vi "Plugin - Mid Measurement.vi"(11 "Message Queues in":T1) -> ()   [LabVIEW 2019]
uses:
  support/Copy of Message Queue/All Message Queues.ctl
  support/Copy of Message Queue/Message Cluster.ctl
  Analysis/Global Tube Measurement.vi
  support/Message Queue/Message Queue.lvlib
  support/Copy of Message Queue/Copy of Message Queue.lvlib
panel:
  in  "Mid Measurement(m)":dbl format="%.4g"
  in  "error in":errorcluster
  out "error out":errorcluster
  in  "Next":bool
  in  "Exit":bool
  # "Enter Mid Measurement"
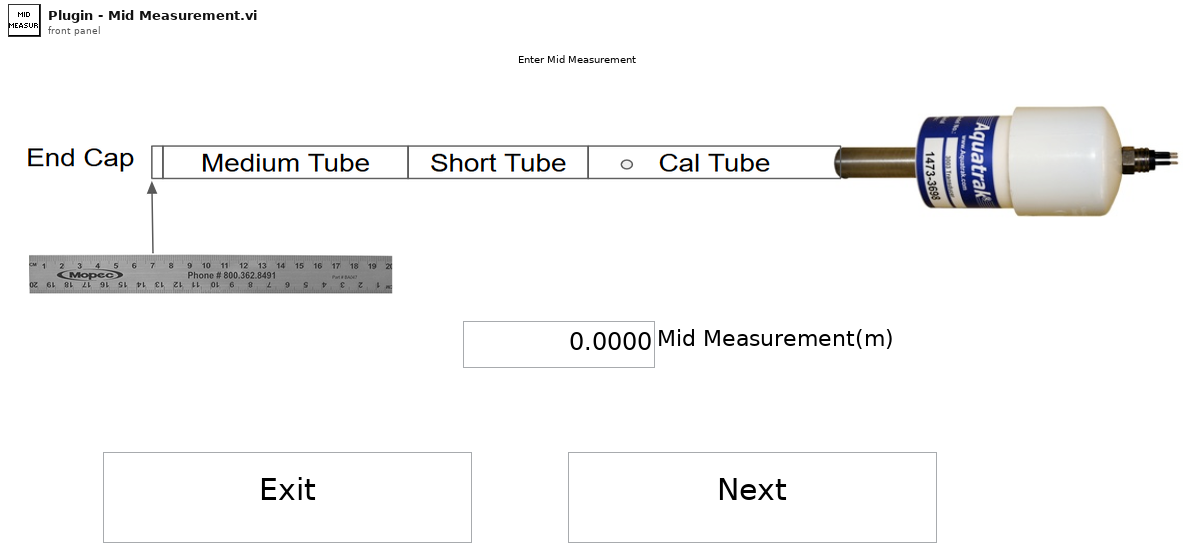
[diagram p1: front panel]
types:
  T1 = typedef "Copy of Message Queue.lvlib/All Message Queues.ctl" = cluster{"UI":refnum<queue>, "Acquisition":refnum<queue>, "Logging":refnum<queue>, "Analyze":refnum<queue>}
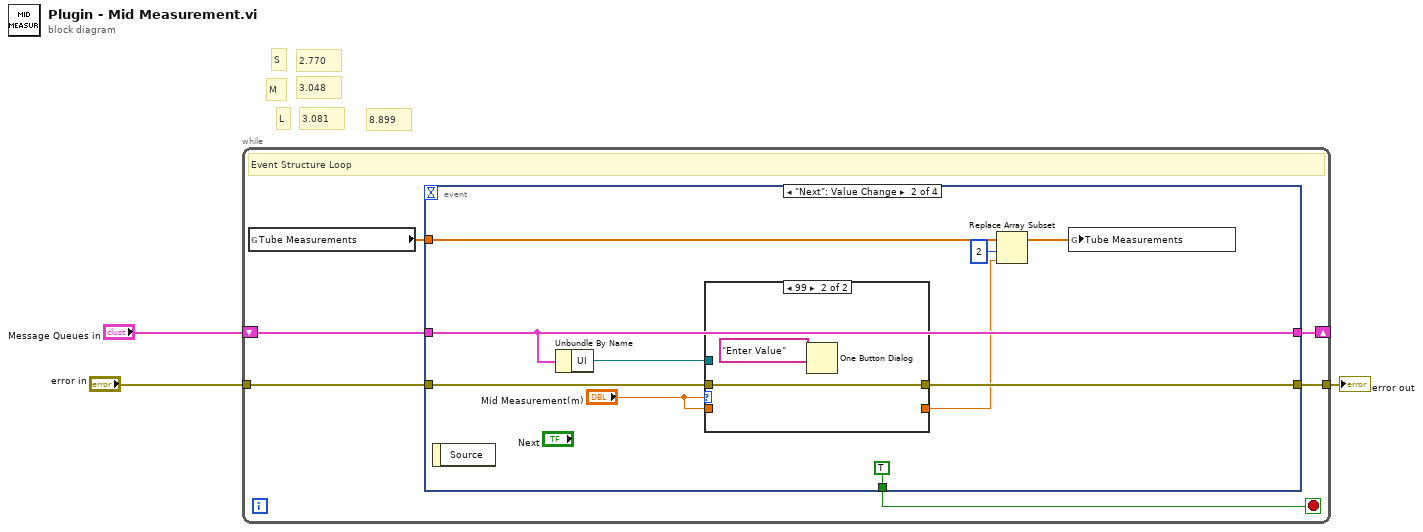
[diagram p0: block diagram]
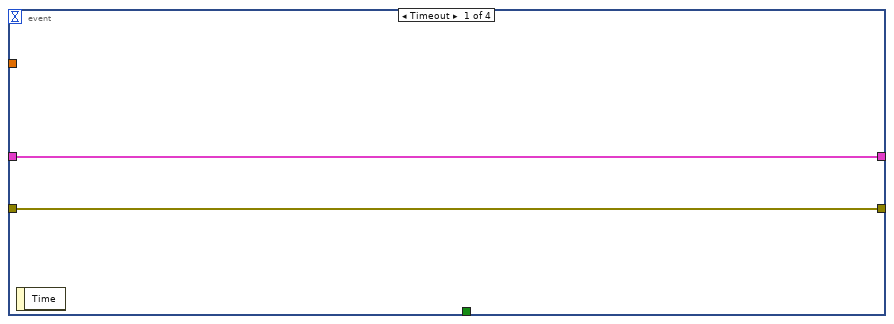
[diagram p2: hidden frame]
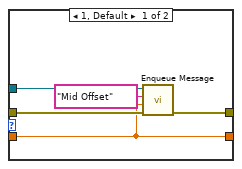
[diagram p3: hidden frame]
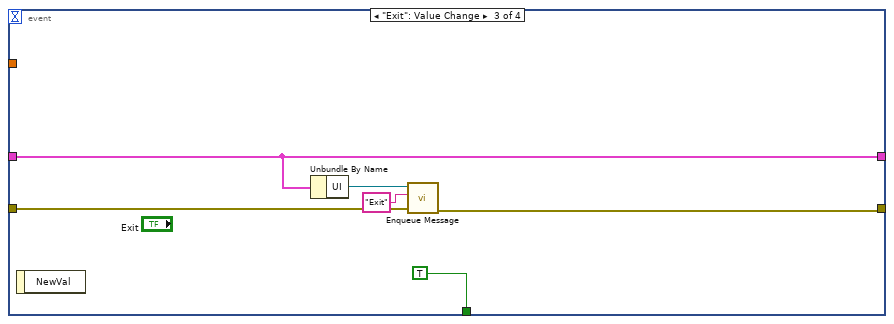
[diagram p4: hidden frame]
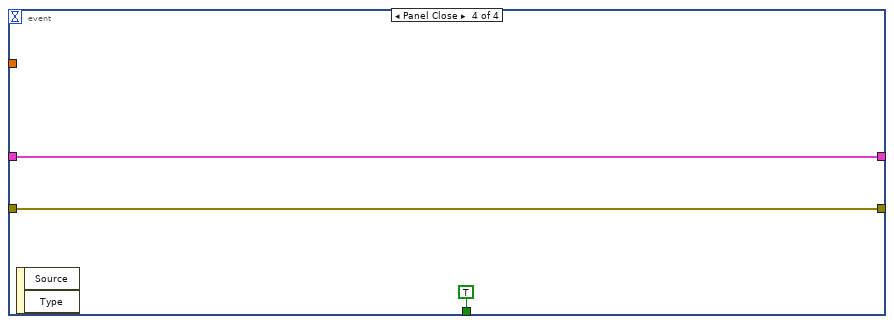
[diagram p5: hidden frame]
diagram:
  # "8.899"
  # "L"
  # "3.081"
  # "M"
  # "S"
  # "2.770"
  # "3.048"
  n1 = while {
    shift-right: [w8] -> _
    shift-left: "Message Queues in" -> [w7]
    tunnel: [w6] -> w2
    tunnel: "error in" -> [w5]
    stop <- w9 stop-if-true
    # "Event Structure Loop"
    n2 = global read "Global Tube Measurement.vi" "Tube Measurements"() -> (w4:dbl[])
    n3 = event shown="[1] \"Next\": Value Change" {
      selector: _ -> [_ _ _ _]
      dyn-events: _ -> [_ _ _ _]
      timeout: _ -> [_ _ _ _]
      tunnel: [_ TRUE ("NewVal") TRUE ("NewVal") TRUE ("NewVal")] -> w9
      tunnel: w7 -> [w11 w21 w31 w37]
      tunnel: [w11 w21 w31 w37] -> w8
      tunnel: [w10 w18 w29 w35] -> w6
      tunnel: w5 -> [w10 w17 w30 w35]
      tunnel: w4 -> [_ w13 _ _]
      event Timeout {
        n4 = event-data() -> ()  [unwired: 1 in, 1 out]
      }
      event "Next": Value Change {
        n5 = event-data() -> ()  [unwired: 1 in, 1 out]
        n6 = Unbundle By Name(w21) -> ("UI"=w20:refnum<queue>)
        n7 = case shown="99" "Mid Measurement(m)" {
          tunnel: w20 -> [w25 _]
          tunnel: [w24 w28] -> w18
          tunnel: w17 -> [w23 w28]
          tunnel: "Mid Measurement(m)" -> [w22 _]
          tunnel: [w22 _] -> w12
          frame 1, Default {
            n8 = call "Enqueue Message.vi"("error in (no error)"=w23, "Message Data"=w22, "Message"="Mid Offset", "Message Queue"=w25) -> ("error out"=w24:errorcluster)  [unwired: 6 in, 1 out]
          }
          frame 99 {
            n9 = One Button Dialog(message="Enter Value") -> ()  [unwired: 1 in, 1 out]
          }
        }
        n10 = Replace Array Subset(array=w13, new element=w12, index=2) -> (w15:dbl[])
        n11 = global write "Global Tube Measurement.vi" "Tube Measurements"(w15) -> ()
      }
      event "Exit": Value Change {
        n12 = event-data() -> ()  [unwired: 1 in, 1 out]
        n13 = Unbundle By Name(w31) -> ("UI"=w32:refnum<queue>)
        n14 = call "Enqueue Message.vi"("error in (no error)"=w30, "Message"="Exit", "Message Queue"=w32) -> ("error out"=w29:errorcluster)  [unwired: 7 in, 1 out]
      }
      event Panel Close {
        n15 = event-data() -> ()  [unwired: 1 in, 2 out]
      }
    }
  }
  "error out" <- w2
